vi "Generate Time Series.vi"() -> (3 "时间序列":dbl[](graph))   [LabVIEW 2012]
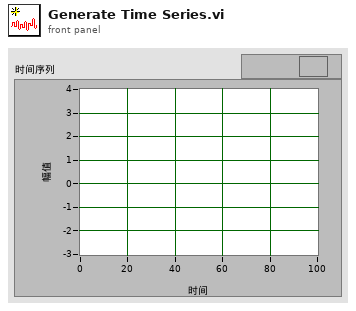
[diagram p1: front panel]
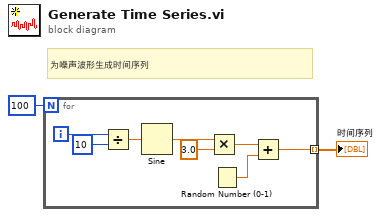
[diagram p0: block diagram]
diagram:
  # "为噪声波形生成时间序列"
  n1 = for "Generate Time Series for Noisy Waveform" {
    N: 100 -> [_]
    tunnel: [w3] -> w1 mode=indexing
    i -> [w10]
    n2 = Divide ("除")(x=w10, y=10) -> (x/y=w9:dbl)
    n3 = Sine ("正弦")(x=w9) -> (sin(x)=w7:dbl)
    n4 = Multiply ("乘")(x=w7, y=3.0) -> (x*y=w5:dbl)
    n5 = Random Number (0-1) ("随机数(0-1)")() -> (number: 0 to 1=w4:dbl)
    n6 = Add ("加")(x=w5, y=w4) -> (x+y=w3:dbl)
  }
  "时间序列" <- w1
